vi "ControlVentTubing (1).vi"(11 "Boolean":bool) -> ()   [LabVIEW 2017]
doc: "Output FALSE to solenoids controlling Levitiation, Suspension, and Magnetic Braking."
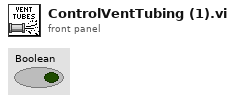
[diagram p1: front panel]
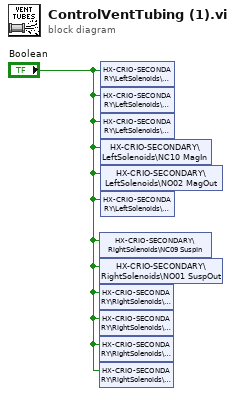
[diagram p0: block diagram]
diagram:
  n1 = shared-variable "HX-CRIO-SECONDARY\\RightSolenoids\\NC09 SuspIn"("Boolean") -> ()  [unwired: 1 in, 1 out]
  n2 = shared-variable "HX-CRIO-SECONDARY\\RightSolenoids\\NO01 SuspOut"("Boolean") -> ()  [unwired: 1 in, 1 out]
  n3 = shared-variable "HX-CRIO-SECONDARY\\RightSolenoids\\NC08"("Boolean") -> ()  [unwired: 1 in, 1 out]
  n4 = shared-variable "HX-CRIO-SECONDARY\\RightSolenoids\\NC05"("Boolean") -> ()  [unwired: 1 in, 1 out]
  n5 = shared-variable "HX-CRIO-SECONDARY\\RightSolenoids\\NC06"("Boolean") -> ()  [unwired: 1 in, 1 out]
  n6 = shared-variable "HX-CRIO-SECONDARY\\RightSolenoids\\NC07"("Boolean") -> ()  [unwired: 1 in, 1 out]
  n7 = shared-variable "HX-CRIO-SECONDARY\\LeftSolenoids\\NC03"("Boolean") -> ()  [unwired: 1 in, 1 out]
  n8 = shared-variable "HX-CRIO-SECONDARY\\LeftSolenoids\\NC04"("Boolean") -> ()  [unwired: 1 in, 1 out]
  n9 = shared-variable "HX-CRIO-SECONDARY\\LeftSolenoids\\NC02"("Boolean") -> ()  [unwired: 1 in, 1 out]
  n10 = shared-variable "HX-CRIO-SECONDARY\\LeftSolenoids\\NC10 MagIn"("Boolean") -> ()  [unwired: 1 in, 1 out]
  n11 = shared-variable "HX-CRIO-SECONDARY\\LeftSolenoids\\NO02 MagOut"("Boolean") -> ()  [unwired: 1 in, 1 out]
  n12 = shared-variable "HX-CRIO-SECONDARY\\LeftSolenoids\\NC01"("Boolean") -> ()  [unwired: 1 in, 1 out]
